vi "LEDStrip(SubVI).vi"(9 "Duty Cycle Red":dbl, 10 "Duty Cycle Green":dbl, 11 "Duty Cycle Blue":dbl) -> ()   [LabVIEW 2017]
uses:
  <vilib>/myRIO/Instrument Drivers/Onboard IO/PWM/typedefs/PWM Configuration.ctl
  <vilib>/myRIO/Instrument Drivers/Onboard IO/PWM/PWM.lvlib
  <vilib>/myRIO/Common/Instrument Driver Framework/myRIO v1.0/PWM/typedefs/PWM Channels Enum.ctl
  <vilib>/myRIO/Common/Instrument Driver Framework/Utilities/typedefs/Generic FPGA Reference.ctl
  <vilib>/myRIO/Common/Instrument Driver Framework/Utilities/typedefs/myRIO v1.0 Reference.ctl
  <vilib>/myRIO/Common/Instrument Driver Framework/Utilities/typedefs/Hardware Version Enum.ctl
  <vilib>/myRIO/Common/Instrument Driver Framework/Utilities/typedefs/myRIO Generic Hardware Reference.ctl
  <vilib>/myRIO/Instrument Drivers/Onboard IO/PWM/typedefs/PWM Reference.ctl
  <vilib>/myRIO/Instrument Drivers/Onboard IO/PWM/vis/Set Duty Cycle and Frequency.vi
  <vilib>/userdefined/High Color/nirio_resource_hc.ctl
  <vilib>/myRIO/Common/Instrument Driver Framework/myRIO v1.0/PWM/vis/myRIO v1.1 Open PWM.vi
  <vilib>/myRIO/Instrument Drivers/Onboard IO/PWM/vis/myRIO PWM Open.xnode
  <vilib>/myRIO/Common/Instrument Driver Framework/Utilities/vis/Is FPGA Ref Available.vi
  <vilib>/myRIO/Express VI/Onboard IO/PWM/PWM Express VI.xnode
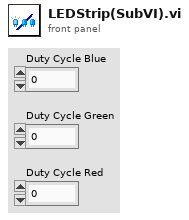
[diagram p1: front panel]
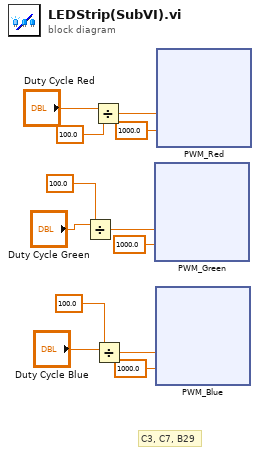
[diagram p0: block diagram]
diagram:
  # "C3, C7, B29"
  n1 = Divide(x="Duty Cycle Green", y=100.0) -> (x/y=w6:dbl)
  n2 = Divide(x="Duty Cycle Red", y=100.0) -> (x/y=w8:dbl)
  n3 = Divide(x="Duty Cycle Blue", y=100.0) -> (x/y=w4:dbl)
  n4 = xnode "PWM_Green"("Duty Cycle"=w6, "Frequency [Hz]"=1000.0) -> ()  [unwired: 1 in, 1 out]
  n5 = xnode "PWM_Blue"("Duty Cycle"=w4, "Frequency [Hz]"=1000.0) -> ()  [unwired: 1 in, 1 out]
  n6 = xnode "PWM_Red"("Duty Cycle"=w8, "Frequency [Hz]"=1000.0) -> ()  [unwired: 1 in, 1 out]
